vi "pf_Execute_Command.vi"(8 "error in (no error)":errorcluster, 10 "Command":string, 11 "IMAQ Session in":refnum<k11>) -> (0 "error out":errorcluster, 3 "IMAQ Session out":refnum<k11>)   [LabVIEW 2025, in "Photonfocus_Toolkit.lvlib"]
doc: "Executes a command."
uses:
  Photonfocus_Toolkit.lvlib
  _Private/Controls/pf_Camera_ctrl_mngr_action.ctl
  _Private/Controls/pf_Toolkit_Error_Type.ctl
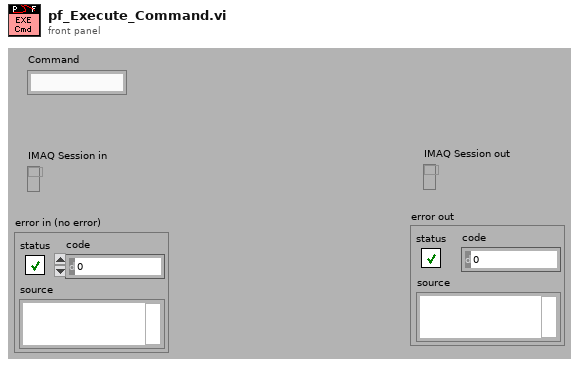
[diagram p1: front panel]
types:
  T1 = typedef "Photonfocus_Toolkit.lvlib/pf_Camera_ctrl_mngr_action.ctl" = enum16{"Create", "Destroy", "Set", "Get"}
  T2 = typedef "Photonfocus_Toolkit.lvlib/pf_Property_Cluster.ctl" = cluster{"Name":string, "Type":T3, "Float.Min":sgl, "Float.Max":sgl, "Float.Value":sgl, "Int.Min":u32, "Int.Max":u32, "Int.Value":u32, "String.Value":string, "MODE.Values":string[], "MODE.Index":i32, "Flag":T4}
  T3 = typedef "Photonfocus_Toolkit.lvlib/pf_Property_Type.ctl" = enum16{"Undefined", "PF_ROOT", "PF_INT", "PF_FLOAT", "PF_BOOL", "PF_MODE", "PF_REGISTER", "PF_STRING", "PF_BUFFER", "PF_STRUCT", "PF_ARRAY", "PF_COMMAND", "PF_EVENT"}
  T4 = typedef "Photonfocus_Toolkit.lvlib/pf_Property_Flag.ctl" = enum16{"Undefined", "RO", "WO", "RW"}
  T5 = typedef "Photonfocus_Toolkit.lvlib/pf_Toolkit_Error_Type.ctl" = enum16{"PF Toolkit_Generic Error", "PF Toolkit_PFConfig Error"}
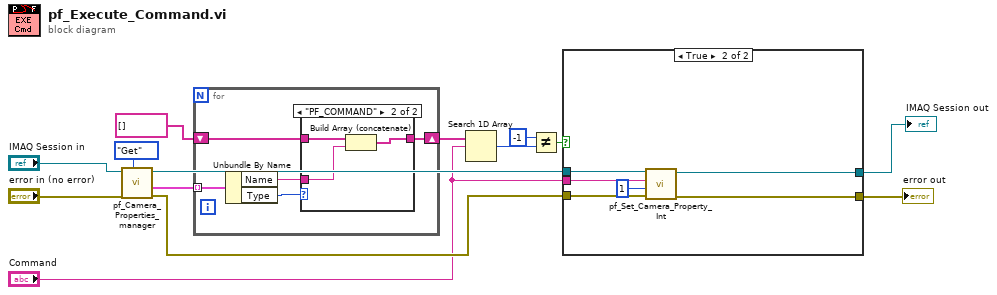
[diagram p0: block diagram]
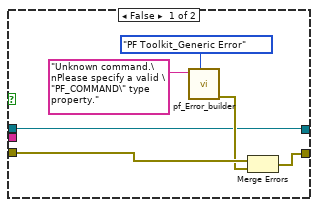
[diagram p2: hidden frame]
diagram:
  n1 = call "pf_Camera_Properties_manager.vi"("Action"=pf_Camera_ctrl_mngr_action."Get", "error in (no error)"="error in (no error)", "IMAQ Session in"="IMAQ Session in") -> ("error out"=w9:errorcluster, "Properties Array out"=w11:T2[], "IMAQ Session out"=w6:refnum<k11>)  [unwired: 2 in, 4 out]
  n2 = for {
    tunnel: w11 -> [w19] mode=indexing
    shift-right: [w15] -> w5
    shift-left: string[] [] -> [w16]
    n3 = Unbundle By Name(w19) -> ("Name"=w17:string, "Type"=w18:T3)
    n4 = case shown="\"PF_COMMAND\"" w18 {
      tunnel: w17 -> [_ w22]
      tunnel: w16 -> [w20 w23]
      tunnel: [w20 w21] -> w15
      frame Default {
      }
      frame "PF_COMMAND" {
        n5 = Build Array (concatenate)(w23, w22) -> (w21:string[])
      }
    }
  }
  n6 = Search 1D Array(1D array=w5, element="Command") -> (index of element=w3:i32)  [unwired: 1 out]
  n7 = Not Equal?(x=-1, y=w3) -> (x != y?=w1:bool)
  n8 = case shown="True" w1 {
    tunnel: [w27 w35] -> w14
    tunnel: [w25 w34] -> w13
    tunnel: w9 -> [w29 w33]
    tunnel: w6 -> [w25 w31]
    tunnel: "Command" -> [_ w30]
    frame False {
      n9 = call "pf_Error_builder.vi"("pf Error Type"=pf_Toolkit_Error_Type."PF Toolkit_Generic Error", "Error message"="Unknown command.\nPlease specify a valid \"PF_COMMAND\" type  property.") -> ("Error cluster out"=w28:errorcluster)  [unwired: 9 out]
      n10 = Merge Errors(w29, w28) -> (w27:errorcluster)
    }
    frame True {
      n11 = call "pf_Set_Camera_Property_Int.vi"("error in (no error)"=w33, "Property Value"=u32 1, "Property Name"=w30, "IMAQ Session in"=w31) -> ("error out"=w35:errorcluster, "IMAQ Session out"=w34:refnum<k11>)  [unwired: 6 out]
    }
  }
  "error out" <- w14
  "IMAQ Session out" <- w13
